vi "Process.vi"(8 "error in":errorcluster, 11 "Measurement.WavelengthSweeping.UI":refnum<class "Measurement.PhotocurrentMapping.UI.lvclass">) -> (0 "error out":errorcluster, 3 "Measurement.WavelengthSweeping.UI out":refnum<class "Measurement.PhotocurrentMapping.UI.lvclass">)   [LabVIEW 2017, in "Measurement.PhotocurrentMapping.UI.lvclass"]
doc: "---------------------------------------------------------------\nJKI State Machine Objects™\nhttp://jki.net/state-machine-objects/\nCopyright (C) 2005-2015, JKI <info@jki.net>\nALL RIGHTS RESERVEDJKI State Machine Objects (SMO) 1.0.0.5\nJKI - JKI\nCopyright (c) 2016, JKI"
uses:
  Measurement.PhotocurrentMapping.UI.lvclass
  D:/Program Files (x86)/National Instruments/LabVIEW 2017/vi.lib/JKI/JKI SMO/SMO/SMO.lvclass
  D:/Program Files (x86)/National Instruments/LabVIEW 2017/vi.lib/JKI/JKI SMO/SMO.UI/SMO.UI.lvclass
  <vilib>/JKI/JKI SMO/SMO/Typedefs/Parent Call--Enum.ctl
  Measurement.PhotocurrentMapping/Typedefs/Measurement.PhotocurrentMapping.Configured--Data.ctl
  Measurement.PhotocurrentMapping/Typedefs/Measurement.PhotocurrentMapping.Measured--Data.ctl
  Typedefs/Grid Data--Cluster.ctl
  Typedefs/Image Data--Cluster.ctl
  Typedefs/Graphs Data--Cluster.ctl
  <vilib>/vision/Image Controls.llb/IMAQ Image.ctl
  Measurement.PhotocurrentMapping/Measurement.PhotocurrentMapping.lvclass
  D:/upwork/Laser Measurement Tool/Laser/project/Subsystems/Measurement/Measurement.lvclass
  Measurement.UI/Measurement.UI.lvclass
  <vilib>/JKI/JKI SMO/SMO/SMO.lvclass
  <vilib>/JKI/JKI SMO/SMO.UI/SMO.UI.lvclass
  Measurement/Measurement.lvclass
panel:
  in  "Clear Button":bool
  in  "Stop Button":bool
  in  "Pause Button":bool
  in  "Start Button":bool
  in  "Close Button":bool
  in  "LIA Auto Scale":bool=TRUE
  in  "SMU Auto Scale":bool=TRUE
  in  "LIA maximum":dbl=1.0 min=0.0 step=0.01 format="%.4f"
  in  "LIA minimum":dbl min=0.0 step=0.01 format="%.4f"
  in  "SMU maximum, A":dbl=1.0 min=0.0 step=0.01 format="%.4f"
  in  "SMU minimum, A":dbl min=0.0 step=0.01 format="%.4f"
  out "Initialized":bool
  out "SMU":T1(plugin-control)
  out "LIA":T1(plugin-control)
  out "SMU":cluster{"X":dbl, "Y":dbl}[](graph) caption="XY Graph - Light"
  out "LIA":cluster{"X":dbl, "Y":dbl}[](graph) caption="XY Graph - Light"
  # "For instructions on how to use the JKI State Machine Objects, examples and video tutorials, visit:\nhttp://jki.net/state-machine-objects/\n\nJKI State Machine Objects™\nhttp://jki.net/state-machine-objects/\nCopyright (C) 2005-2015, JKI <info@jki.net>\nALL RIGHTS RESERVED"
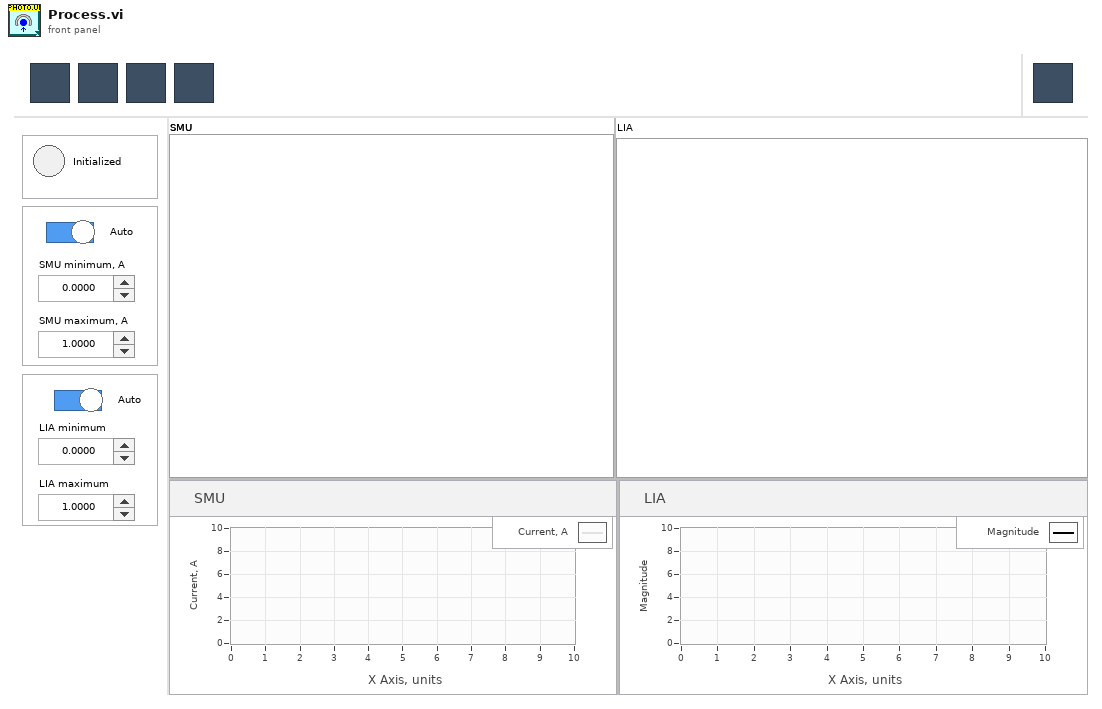
[diagram p1: front panel]
types:
  T1 = typedef "IMAQ Image.ctl" = refnum<image>
  T2 = typedef "SMO.lvclass/Parent Call--Enum.ctl" = enum16{"Allows parent to run", "Does not request parent to run"}
  T3 = enum8{"Enabled", "Disabled", "Disabled and Grayed Out"}
  T4 = enum32{"invalid app kind", "Development System", "Run Time System", "Student Edition", "Embedded LabVIEW", "Evaluation", "Custom"}
  T5 = enum32{"Invalid", "Standard", "Closed", "Hidden", "Minimized", "Maximized"}
  T6 = typedef "Measurement.lvclass/PublicEvents--Measurement.Initialized.ctl" = bool
  T7 = typedef "Measurement.PhotocurrentMapping.lvclass/Measurement.PhotocurrentMapping.Configured--Data.ctl" = cluster{"X Count":i32, "Y Count":i32}
  T8 = typedef "Measurement.lvclass/PublicEvents--Measurement.Configured.ctl" = variant
  T9 = typedef "Measurement.PhotocurrentMapping.UI.lvclass/Dependencies--Cluster.ctl" = cluster{"Measurement.PhotocurrentMapping":refnum<class "Measurement.PhotocurrentMapping.lvclass">}
  T10 = typedef "Measurement.PhotocurrentMapping.lvclass/Measurement.PhotocurrentMapping.Measured--Data.ctl" = cluster{"X Value, units":dbl, "Y Value, units":dbl, "X Index":i32, "Y Index":i32, "Current, A":dbl, "Magnitude":dbl, "Last Row Element?":bool}
  T11 = typedef "Measurement.PhotocurrentMapping.UI.lvclass/Grid Data--Cluster.ctl" = cluster{"SMU Image":T12, "LIA Image":T12, "Filled Row":i32}
  T12 = typedef "Measurement.PhotocurrentMapping.UI.lvclass/Image Data--Cluster.ctl" = cluster{"Raw":dbl[][], "Normalized":dbl[][], "Minimum":dbl, "Maximum":dbl}
  T13 = typedef "Measurement.PhotocurrentMapping.UI.lvclass/Graphs Data--Cluster.ctl" = cluster{"SMU Data":cluster{"X":dbl, "Y":dbl}[], "LIA Data":cluster{"X":dbl, "Y":dbl}[], "SMU Buffer":cluster{"X":dbl, "Y":dbl}[], "LIA Buffer":cluster{"X":dbl, "Y":dbl}[]}
  T14 = cluster{"Core":cluster{"Current VI Reference":refnum<vi>, "Close Panel on Exit?":bool, "error":errorcluster}, "Self Reference":refnum<class "Measurement.PhotocurrentMapping.UI.lvclass">, "Dependencies":T9, "Measured":T10, "X Count":i32, "Y Count":i32, "Grid Data":T11, "Graphs Data":T13, "SMU Image":T1, "LIA Image":T1}
  T15 = typedef "Measurement.lvclass/PublicEvents--Measurement.Measured.ctl" = variant
  T16 = typedef "Measurement.lvclass/PublicEvents--Measurement.Finished.ctl" = bool
  T17 = cluster{"Current VI Reference":refnum<vi>, "Close Panel on Exit?":bool, "error":errorcluster}
  T18 = typedef "Image Type" = u32
  T19 = typedef "SMO.lvclass/Protected Events.ctl" = cluster{"StopProcesses":refnum<user-event>, "AbortProcesses":refnum<user-event>, "Config Changed":refnum<user-event>, "Dependency":refnum<user-event>}
  T20 = cluster{"Event Registration Refnum":refnum<event-registration>, "Measurement Public Events":refnum<event-registration>}
  T21 = cluster{"X Value, units":dbl, "Current, A":dbl}[]
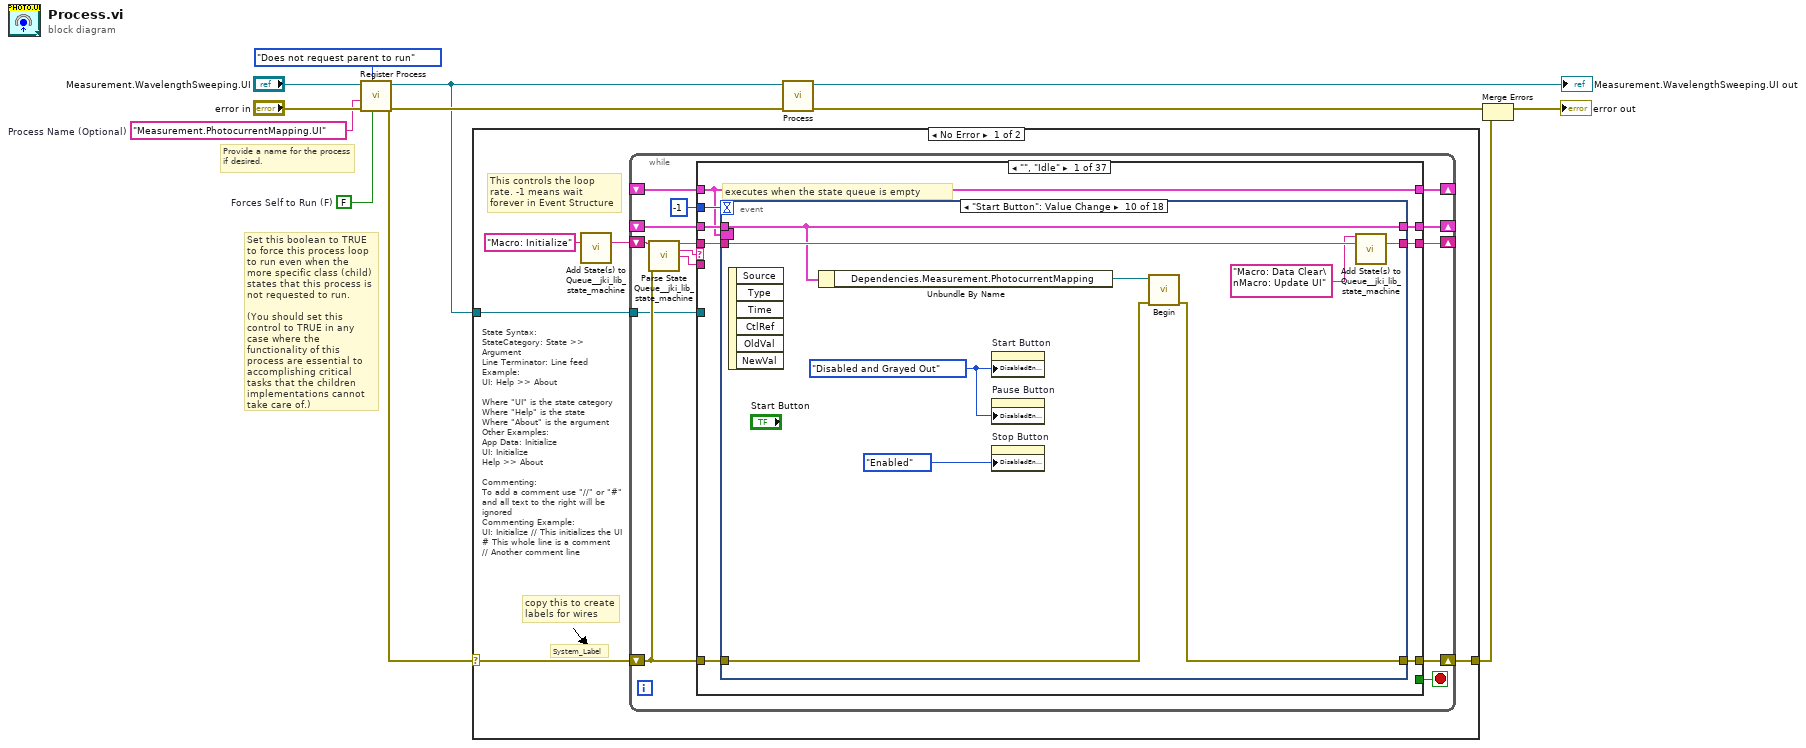
[diagram p0: block diagram]
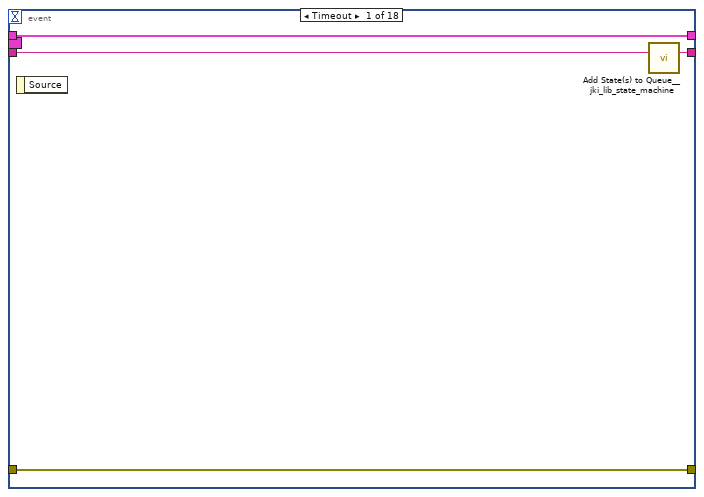
[diagram p2: hidden frame]
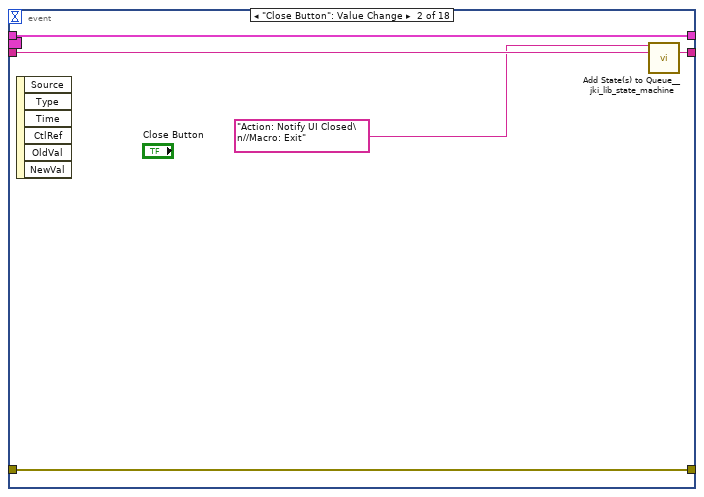
[diagram p3: hidden frame]
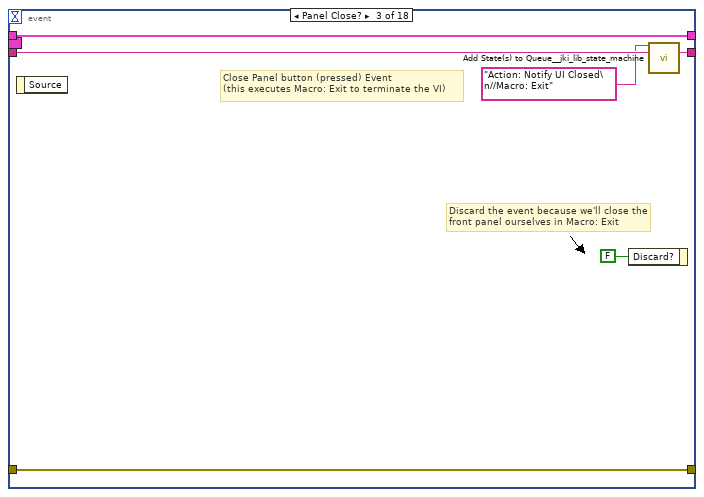
[diagram p4: hidden frame]
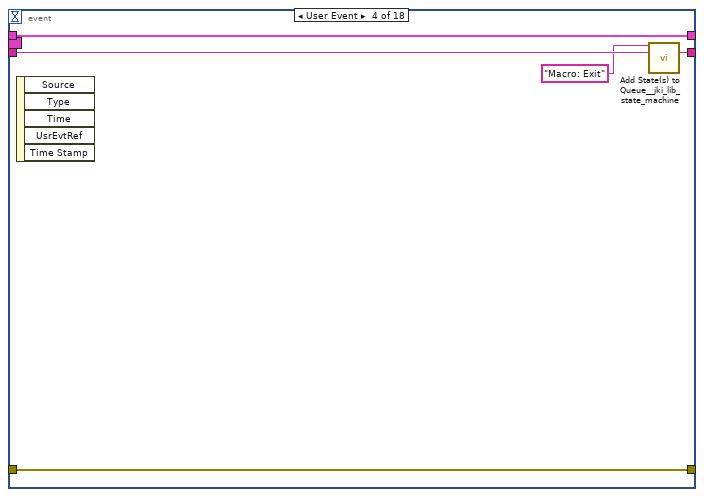
[diagram p5: hidden frame]
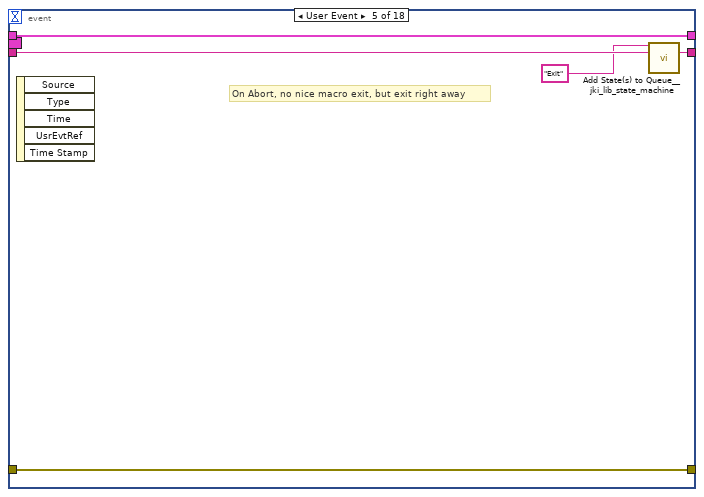
[diagram p6: hidden frame]
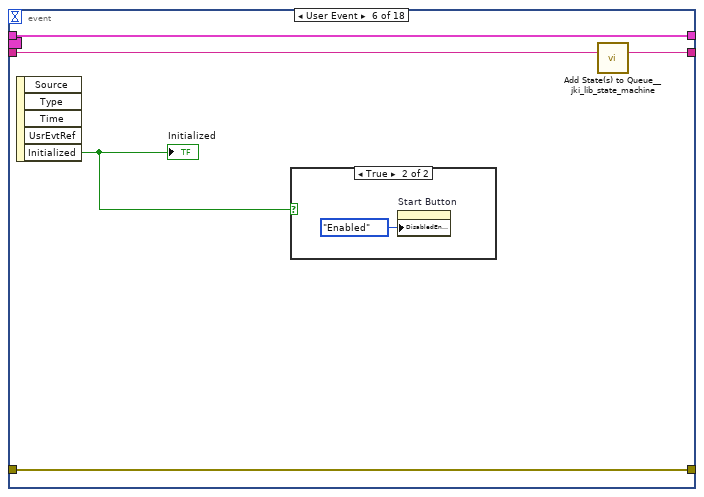
[diagram p7: hidden frame]
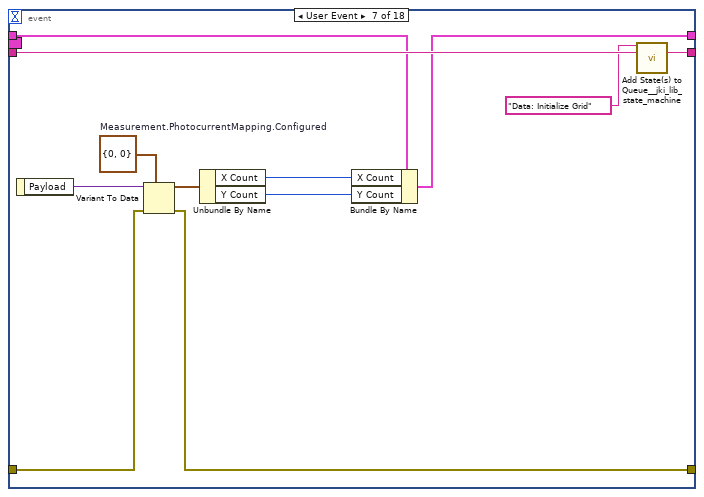
[diagram p9: hidden frame]
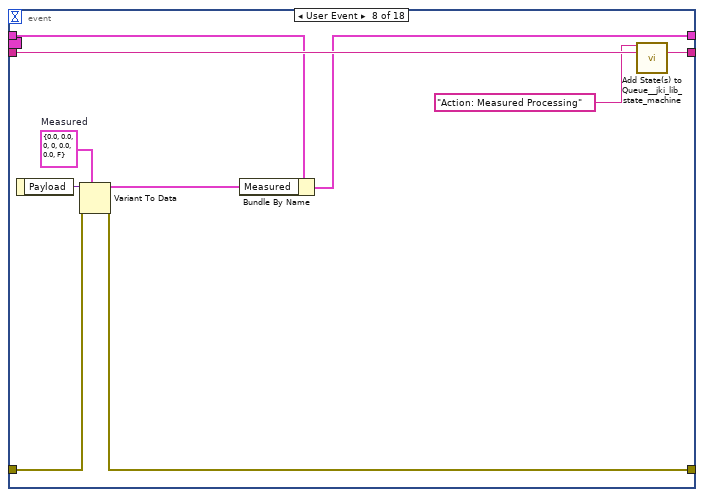
[diagram p10: hidden frame]
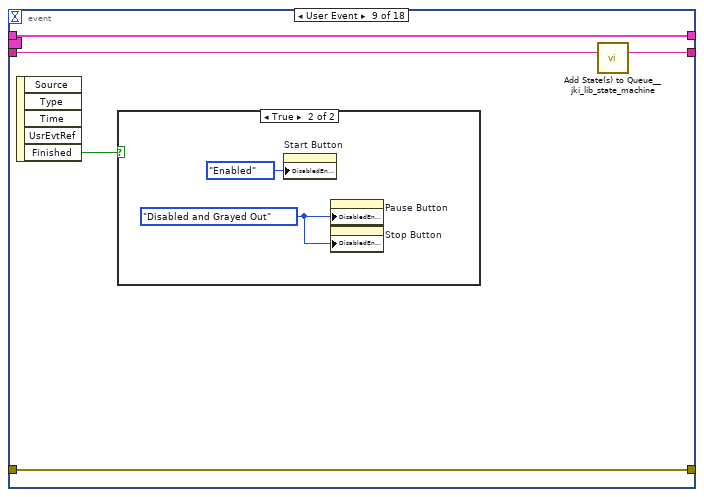
[diagram p11: hidden frame]
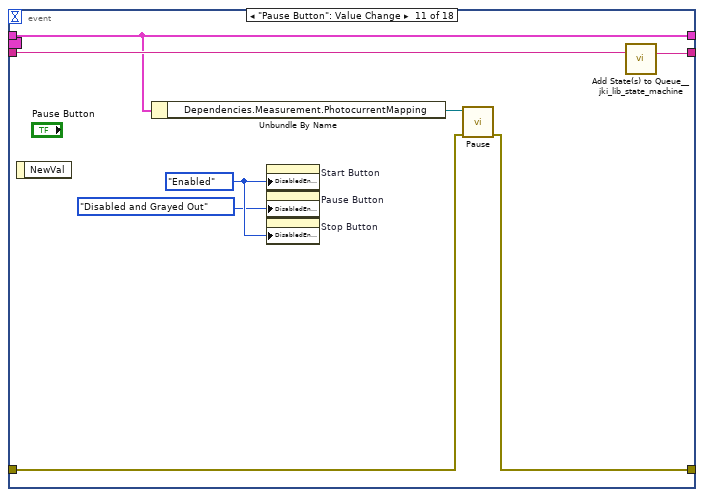
[diagram p13: hidden frame]
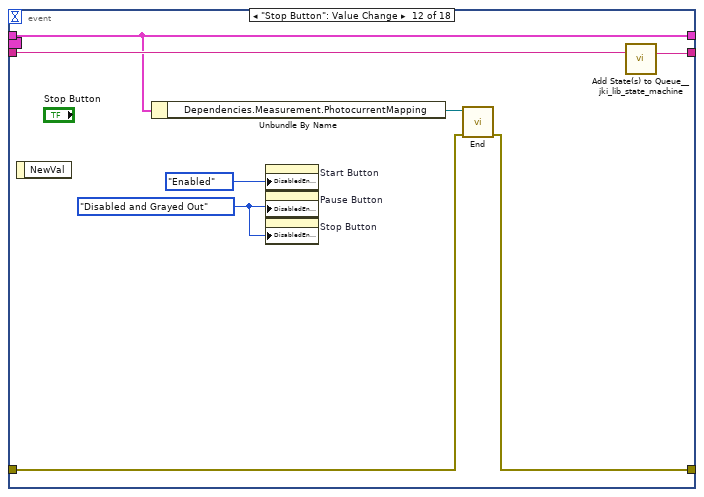
[diagram p14: hidden frame]
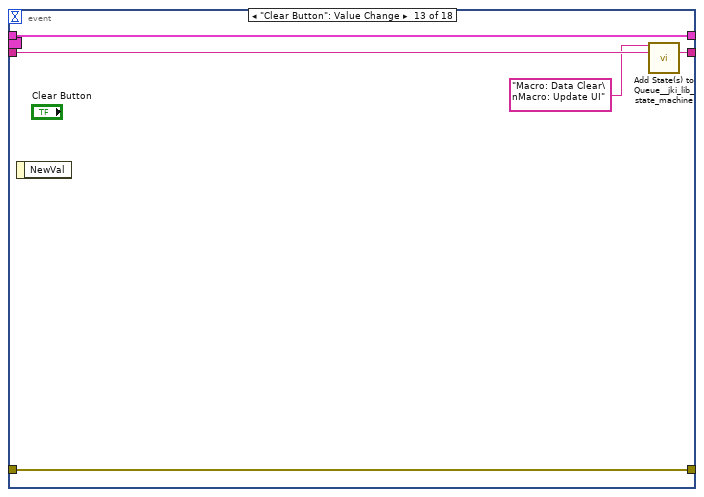
[diagram p15: hidden frame]
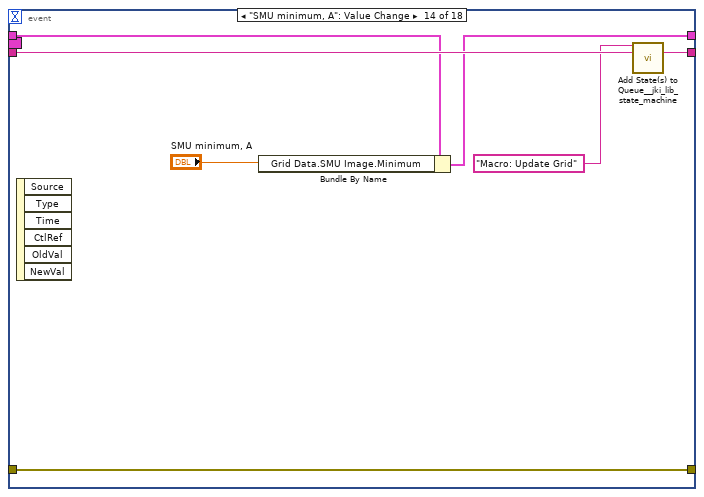
[diagram p16: hidden frame]
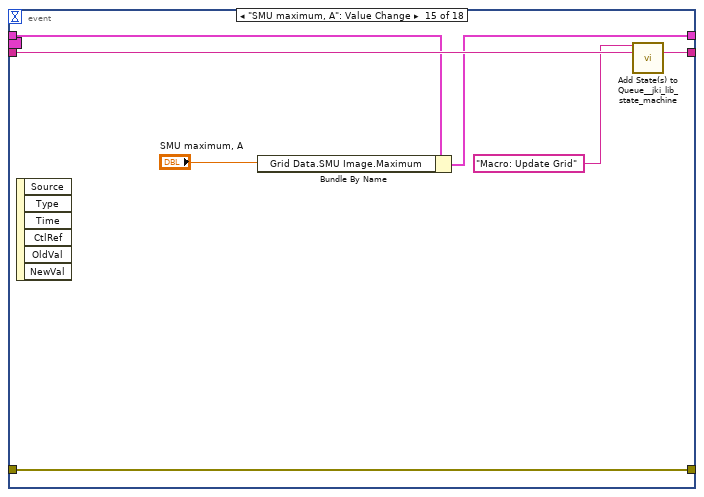
[diagram p17: hidden frame]
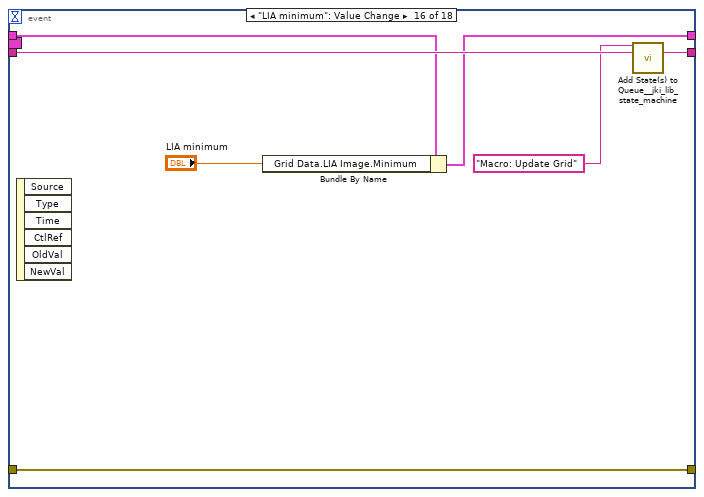
[diagram p18: hidden frame]
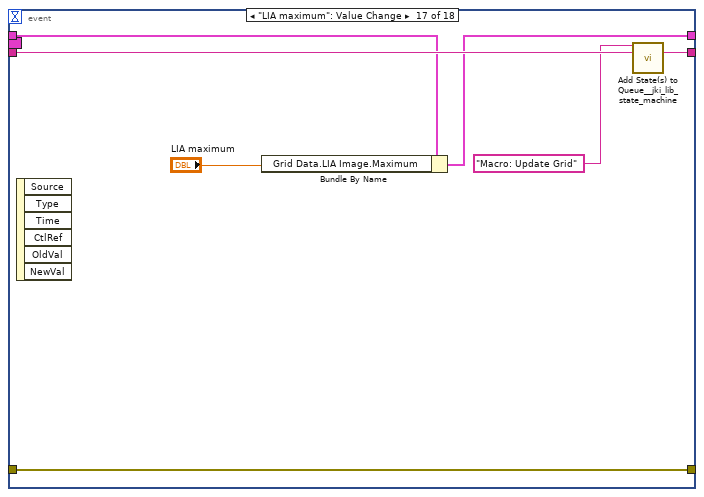
[diagram p19: hidden frame]
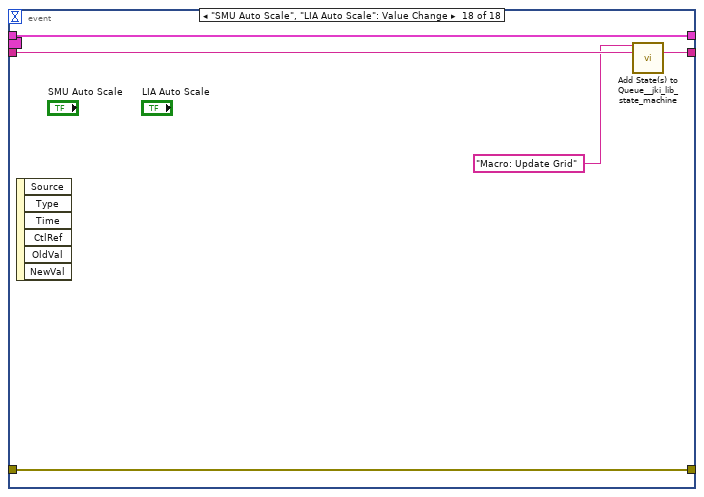
[diagram p20: hidden frame]
diagram:
  w2 = FALSE  # Forces Self to Run (F)
  w1 = "Measurement.PhotocurrentMapping.UI"  # Process Name (Optional)
  # "Provide a name for the process\nif desired."
  # "Set this boolean to TRUE to force this process loop to run even when the more specific class (child) states that this process is not requested to run.\n\n(You should set this control to TRUE in any case where the functionality of this process are essential to accomplishing critical tasks that the children implementations cannot take care of.)"
  n1 = call <vilib>:"Register Process.vi"("Forces Self to Run (F)"=w2, "Parent Call"=Parent_Call--Enum."Does not request parent to run", "error in (no error)"="error in", "Process Name (optional)"=w1, "SMO"="Measurement.WavelengthSweeping.UI") -> ("error out"=w8:errorcluster, "SMO out"=w7:refnum<class "Measurement.PhotocurrentMapping.UI.lvclass">)  [unwired: 5 in]
  n2 = case shown="No Error" w8 {
    selector: w8 -> [w13 w573]
    tunnel: w7 -> [w14 _]
    tunnel: [w12 w573] -> w4
    frame No Error {
      # "State Syntax:\nStateCategory: State >> Argument\nLine Terminator: Line feed\nExample:\nUI: Help >> About\n\nWhere \"UI\" is the state category\nWhere \"Help\" is the state\nWhere \"About\" is the argument\nOther Examples:\nApp Data: Initialize\nUI: Initialize\nHelp >> About\n\nCommenting:\nTo add a comment use \"//\" or \"#\" and all text to the right will be ignored\nCommenting Example:\nUI: Initialize // This initializes the UI\n# This whole line is a comment\n// Another comment line"
      # "copy this to create labels for wires"
      # "This controls the loop rate. -1 means wait forever in Event Structure"
      # "System_Label"
      n3 = call <vilib>:"Add State(s) to Queue__jki_lib_state_machine.vi"("State(s) in (\"\")"="Macro: Initialize") -> ("States Out"=w16:string)  [unwired: 14 in]
      n4 = while {
        shift-right: [w23] -> _
        shift-left: _ -> [w22]
        shift-right: [w26] -> w12
        shift-left: w13 -> [w20]
        shift-right: [w25] -> _
        shift-left: w16 -> [w27]
        tunnel: w14 -> [w19]
        shift-right: [w18] -> _
        shift-left: _ -> [w17]
        stop <- w24 stop-if-true
        n5 = call <vilib>:"Parse State Queue__jki_lib_state_machine.vi"("State Queue"=w27, "Error In (no error)"=w20) -> ("Remaining States"=w29:string, "Current State"=w30:string, "Arguments"=w28:string)  [unwired: 11 in]
        n6 = case shown="\"\", \"Idle\"" w30 {
          selector: w30 -> [_ _ w168 _ _ _ _ _ _ _ _ _ _ _ _ _ _ _ _ _ _ _ _ _ _ _ _ _ _ _ _ _ _ _ _ _ _]
          tunnel: w29 -> [w38 w166 w172 w191 w205 w211 w216 w235 w242 w253 w259 w272 w277 w292 w299 w315 w349 w356 w361 w370 w384 w390 w396 w402 w407 w418 w423 w437 w443 w450 w457 w463 w481 w512 w527 w557 w572]
          tunnel: w28 -> [_ _ _ _ _ _ _ _ _ _ _ _ _ _ w293 w309 _ _ _ _ _ _ _ _ _ _ _ _ _ _ _ _ _ _ _ _ _]
          tunnel: w22 -> [w36 w163 w170 w182 w194 w207 w213 _ w237 w247 w257 w266 w274 w288 w297 w311 w345 w352 w358 w366 w375 w387 w393 w399 w404 w415 w420 w429 w441 w446 w453 w458 w476 w507 w518 w542 w563]
          tunnel: [w35 w164 w174 w188 w196 w206 w214 w224 w238 w250 w258 w269 w275 w278 w294 w312 w346 w353 w359 w368 w382 w388 w394 w400 w405 w409 w421 w431 w438 w447 w451 w460 w478 w509 w524 w554 w560] -> w26
          tunnel: w20 -> [w34 w164 w173 w188 w201 _ w214 w232 w239 w250 w258 w269 w275 w280 w295 w313 w346 w353 w359 w368 w382 w388 w394 w400 w405 w410 w421 w433 w439 w447 w452 w460 w478 w509 w524 w554 w561]
          tunnel: [w37 w165 w171 w190 w204 w210 w215 w234 w241 w252 w260 w271 w276 w291 w298 w314 w348 w355 w360 w369 w383 w389 w395 w401 w406 w417 w422 w436 w442 w449 w456 w462 w480 w511 w526 w556 w571] -> w25
          tunnel: [_ _ _ _ _ TRUE _ _ _ _ _ _ _ _ _ _ _ _ _ _ _ _ _ _ _ _ _ _ _ _ _ _ _ _ _ _ _] -> w24
          tunnel: [w33 w163 w170 w189 w193 w207 w213 w233 w237 w246 w256 w265 w274 w287 w297 w311 w345 w352 w358 w366 w375 w387 w393 w399 w404 w415 w420 w429 w441 w445 w453 w458 w475 w506 w523 w553 w566] -> w23
          tunnel: -1 ("Timeout") -> [w32 _ _ _ _ _ _ _ _ _ _ _ _ _ _ _ _ _ _ _ _ _ _ _ _ _ _ _ _ _ _ _ _ _ _ _ _]
          tunnel: w19 -> [_ _ _ _ _ _ _ w230 _ _ _ _ _ _ _ _ _ _ _ _ _ _ _ _ _ _ _ _ _ _ _ _ _ _ _ _ _]
          tunnel: [w31 w162 w167 w179 w203 w208 w212 w229 w236 w251 w261 w270 w273 w290 w296 w308 w347 w354 w357 w367 w376 w386 w392 w398 w403 w416 w419 w426 w440 w448 w455 w461 w479 w510 w525 w555 w570] -> w18
          tunnel: w17 -> [w31 w162 w167 w179 w203 w208 w212 w229 w236 w251 w261 w270 w273 w290 w296 w308 w347 w354 w357 w367 w376 w386 w392 w398 w403 w416 w419 _ w440 w448 w455 w461 w479 w510 w525 w555 w570]
          frame "", "Idle" {
            # "executes when the state queue is empty"
            n7 = event shown="[9] \"Start Button\": Value Change" {
              selector: w31 -> [_ _ _ _ _ _ _ _ _ _ _ _ _ _ _ _ _ _]
              dyn-events: _ -> [_ _ _ _ _ _ _ _ _ _ _ _ _ _ _ _ _ _]
              timeout: w32 -> [_ _ _ _ _ _ _ _ _ _ _ _ _ _ _ _ _ _]
              tunnel: w38 -> [w42 w47 w53 w58 w63 w65 w80 w90 w93 w106 w114 w122 w128 w133 w140 w147 w154 w159]
              tunnel: [w41 w46 w52 w57 w62 w66 w81 w91 w94 w107 w115 w123 w127 w134 w141 w148 w155 w160] -> w37
              tunnel: w36 -> [w39 w44 w49 w55 w60 w67 w74 w84 w95 w105 w113 w121 w125 w132 w139 w146 w153 w158]
              tunnel: [w40 w45 w48 w56 w61 w68 w78 w85 w96 w102 w110 w118 w126 w135 w142 w149 w156 w161] -> w35
              tunnel: w34 -> [w40 w45 w48 w56 w61 w68 w79 w89 w96 w103 w111 w119 w126 w135 w142 w149 w156 w161]
              tunnel: [w39 w44 w49 w55 w60 w67 w73 w83 w95 w105 w113 w121 w125 w131 w138 w145 w152 w158] -> w33
              event Timeout {
                n8 = event-data() -> ()  [unwired: 1 in, 1 out]
                n9 = call <vilib>:"Add State(s) to Queue__jki_lib_state_machine.vi"("State(s) in (\"\")"=w42) -> ("States Out"=w41:string)  [unwired: 14 in]
              }
              event "Close Button": Value Change {
                n10 = event-data() -> ()  [unwired: 1 in, 6 out]
                n11 = call <vilib>:"Add State(s) to Queue__jki_lib_state_machine.vi"("State(s) in Front (\"\")"="Action: Notify UI Closed\n//Macro: Exit" ("State(s) in Front (\"\")"), "State(s) in (\"\")"=w47) -> ("States Out"=w46:string)  [unwired: 13 in]
              }
              event Panel Close? {
                # "Discard the event because we'll close the front panel ourselves in Macro: Exit"
                # "Close Panel button (pressed) Event\n(this executes Macro: Exit to terminate the VI)"
                n12 = event-data() -> ()  [unwired: 1 in, 1 out]
                n13 = event-data("Discard?"=FALSE) -> ()  [unwired: 1 in, 1 out]
                n14 = call <vilib>:"Add State(s) to Queue__jki_lib_state_machine.vi"("State(s) in Front (\"\")"="Action: Notify UI Closed\n//Macro: Exit", "State(s) in (\"\")"=w53) -> ("States Out"=w52:string)  [unwired: 13 in]
              }
              event User Event {
                n15 = event-data() -> ()  [unwired: 1 in, 5 out]
                n16 = call <vilib>:"Add State(s) to Queue__jki_lib_state_machine.vi"("State(s) in Front (\"\")"="Macro: Exit", "State(s) in (\"\")"=w58) -> ("States Out"=w57:string)  [unwired: 13 in]
              }
              event User Event {
                # "On Abort, no nice macro exit, but exit right away"
                n17 = event-data() -> ()  [unwired: 1 in, 5 out]
                n18 = call <vilib>:"Add State(s) to Queue__jki_lib_state_machine.vi"("State(s) in Front (\"\")"="Exit", "State(s) in (\"\")"=w63) -> ("States Out"=w62:string)  [unwired: 13 in]
              }
              event User Event {
                n19 = event-data() -> ("Initialized"=w64:T6)  [unwired: 1 in, 4 out]
                "Initialized" <- w64
                n20 = case shown="True" w64 {
                  frame False {
                  }
                  frame True {
                    n21 = property on="Start Button" class="Bool"("DisabledEnum"=T3."Enabled" ("Disabled")) -> ()  [unwired: 2 in, 2 out]
                  }
                }
                n22 = call <vilib>:"Add State(s) to Queue__jki_lib_state_machine.vi"("State(s) in (\"\")"=w65) -> ("States Out"=w66:string)  [unwired: 14 in]
              }
              event User Event {
                w76 = T7 {"X Count"=0, "Y Count"=0}  # Measurement.PhotocurrentMapping.Configured
                n23 = event-data() -> ("Payload"=w77:T8)  [unwired: 1 in]
                n24 = Variant To Data(error in=w79, type=w76, Variant=w77) -> (data=w75:T7, error out=w78:errorcluster)
                n25 = Unbundle By Name(w75) -> ("X Count"=w72:i32, "Y Count"=w71:i32)
                n26 = Bundle By Name(cluster=w74, "X Count"=w72, "Y Count"=w71) -> (w73:T14)
                n27 = call <vilib>:"Add State(s) to Queue__jki_lib_state_machine.vi"("State(s) in Front (\"\")"="Data: Initialize Grid", "State(s) in (\"\")"=w80) -> ("States Out"=w81:string)  [unwired: 13 in]
              }
              event User Event {
                w87 = T10 {"X Value, units"=0.0, "Y Value, units"=0.0, "X Index"=0, "Y Index"=0, "Current, A"=0.0, "Magnitude"=0.0, "Last Row Element?"=FALSE}  # Measured
                n28 = event-data() -> ("Payload"=w88:T15)  [unwired: 1 in]
                n29 = Variant To Data(error in=w89, type=w87, Variant=w88) -> (data=w82:T10, error out=w85:errorcluster)
                n30 = Bundle By Name(cluster=w84, "Measured"=w82) -> (w83:T14)
                n31 = call <vilib>:"Add State(s) to Queue__jki_lib_state_machine.vi"("State(s) in Front (\"\")"="Action: Measured Processing", "State(s) in (\"\")"=w90) -> ("States Out"=w91:string)  [unwired: 13 in]
              }
              event User Event {
                n32 = event-data() -> ("Finished"=w92:T16)  [unwired: 1 in, 4 out]
                n33 = case shown="True" w92 {
                  frame False {
                  }
                  frame True {
                    w97 = T3."Disabled and Grayed Out" ("Disabled")
                    n34 = property on="Start Button" class="Bool"("DisabledEnum"=T3."Enabled" ("Disabled")) -> ()  [unwired: 2 in, 2 out]
                    n35 = property on="Pause Button" class="Bool"("DisabledEnum"=w97) -> ()  [unwired: 2 in, 2 out]
                    n36 = property on="Stop Button" class="Bool"("DisabledEnum"=w97) -> ()  [unwired: 2 in, 2 out]
                  }
                }
                n37 = call <vilib>:"Add State(s) to Queue__jki_lib_state_machine.vi"("State(s) in (\"\")"=w93) -> ("States Out"=w94:string)  [unwired: 14 in]
              }
              event "Start Button": Value Change {
                w100 = T3."Disabled and Grayed Out" ("Disabled")
                n38 = event-data() -> ()  [unwired: 1 in, 6 out]
                n39 = Unbundle By Name(w105) -> ("Dependencies.Measurement.PhotocurrentMapping"=w104:refnum<class "Measurement.PhotocurrentMapping.lvclass">)
                n40 = property on="Start Button" class="Bool"("DisabledEnum"=w100) -> ()  [unwired: 2 in, 2 out]
                n41 = property on="Pause Button" class="Bool"("DisabledEnum"=w100) -> ()  [unwired: 2 in, 2 out]
                n42 = property on="Stop Button" class="Bool"("DisabledEnum"=T3."Enabled" ("Disabled")) -> ()  [unwired: 2 in, 2 out]
                n43 = call "Begin.vi"("error in (no error)"=w103, "Measurement in"=w104) -> ("error out"=w102:errorcluster)  [unwired: 8 in, 1 out]
                n44 = call <vilib>:"Add State(s) to Queue__jki_lib_state_machine.vi"("State(s) in Front (\"\")"="Macro: Data Clear\nMacro: Update UI", "State(s) in (\"\")"=w106) -> ("States Out"=w107:string)  [unwired: 13 in]
              }
              event "Pause Button": Value Change {
                w109 = T3."Enabled" ("Disabled")
                n45 = event-data() -> ()  [unwired: 1 in, 1 out]
                n46 = Unbundle By Name(w113) -> ("Dependencies.Measurement.PhotocurrentMapping"=w112:refnum<class "Measurement.PhotocurrentMapping.lvclass">)
                n47 = property on="Start Button" class="Bool"("DisabledEnum"=w109) -> ()  [unwired: 2 in, 2 out]
                n48 = property on="Pause Button" class="Bool"("DisabledEnum"=T3."Disabled and Grayed Out" ("Disabled")) -> ()  [unwired: 2 in, 2 out]
                n49 = property on="Stop Button" class="Bool"("DisabledEnum"=w109) -> ()  [unwired: 2 in, 2 out]
                n50 = call "Pause.vi"("error in (no error)"=w111, "Measurement in"=w112) -> ("error out"=w110:errorcluster)  [unwired: 8 in, 1 out]
                n51 = call <vilib>:"Add State(s) to Queue__jki_lib_state_machine.vi"("State(s) in (\"\")"=w114) -> ("States Out"=w115:string)  [unwired: 14 in]
              }
              event "Stop Button": Value Change {
                w116 = T3."Disabled and Grayed Out" ("Disabled")
                n52 = event-data() -> ()  [unwired: 1 in, 1 out]
                n53 = Unbundle By Name(w121) -> ("Dependencies.Measurement.PhotocurrentMapping"=w120:refnum<class "Measurement.PhotocurrentMapping.lvclass">)
                n54 = property on="Start Button" class="Bool"("DisabledEnum"=T3."Enabled" ("Disabled")) -> ()  [unwired: 2 in, 2 out]
                n55 = property on="Pause Button" class="Bool"("DisabledEnum"=w116) -> ()  [unwired: 2 in, 2 out]
                n56 = property on="Stop Button" class="Bool"("DisabledEnum"=w116) -> ()  [unwired: 2 in, 2 out]
                n57 = call "End.vi"("error in (no error)"=w119, "Measurement in"=w120) -> ("error out"=w118:errorcluster)  [unwired: 8 in, 1 out]
                n58 = call <vilib>:"Add State(s) to Queue__jki_lib_state_machine.vi"("State(s) in (\"\")"=w122) -> ("States Out"=w123:string)  [unwired: 14 in]
              }
              event "Clear Button": Value Change {
                n59 = event-data() -> ()  [unwired: 1 in, 1 out]
                n60 = call <vilib>:"Add State(s) to Queue__jki_lib_state_machine.vi"("State(s) in Front (\"\")"="Macro: Data Clear\nMacro: Update UI", "State(s) in (\"\")"=w128) -> ("States Out"=w127:string)  [unwired: 13 in]
              }
              event "SMU minimum, A": Value Change {
                n61 = event-data() -> ()  [unwired: 1 in, 6 out]
                n62 = Bundle By Name(cluster=w132, "Grid Data.SMU Image.Minimum"="SMU minimum, A") -> (w131:T14)
                n63 = call <vilib>:"Add State(s) to Queue__jki_lib_state_machine.vi"("State(s) in Front (\"\")"="Macro: Update Grid" ("State(s) in Front (\"\")"), "State(s) in (\"\")"=w133) -> ("States Out"=w134:string)  [unwired: 13 in]
              }
              event "SMU maximum, A": Value Change {
                n64 = event-data() -> ()  [unwired: 1 in, 6 out]
                n65 = Bundle By Name(cluster=w139, "Grid Data.SMU Image.Maximum"="SMU maximum, A") -> (w138:T14)
                n66 = call <vilib>:"Add State(s) to Queue__jki_lib_state_machine.vi"("State(s) in Front (\"\")"="Macro: Update Grid" ("State(s) in Front (\"\")"), "State(s) in (\"\")"=w140) -> ("States Out"=w141:string)  [unwired: 13 in]
              }
              event "LIA minimum": Value Change {
                n67 = event-data() -> ()  [unwired: 1 in, 6 out]
                n68 = Bundle By Name(cluster=w146, "Grid Data.LIA Image.Minimum"="LIA minimum") -> (w145:T14)
                n69 = call <vilib>:"Add State(s) to Queue__jki_lib_state_machine.vi"("State(s) in Front (\"\")"="Macro: Update Grid" ("State(s) in Front (\"\")"), "State(s) in (\"\")"=w147) -> ("States Out"=w148:string)  [unwired: 13 in]
              }
              event "LIA maximum": Value Change {
                n70 = event-data() -> ()  [unwired: 1 in, 6 out]
                n71 = Bundle By Name(cluster=w153, "Grid Data.LIA Image.Maximum"="LIA maximum") -> (w152:T14)
                n72 = call <vilib>:"Add State(s) to Queue__jki_lib_state_machine.vi"("State(s) in Front (\"\")"="Macro: Update Grid" ("State(s) in Front (\"\")"), "State(s) in (\"\")"=w154) -> ("States Out"=w155:string)  [unwired: 13 in]
              }
              event "SMU Auto Scale", "LIA Auto Scale": Value Change {
                n73 = event-data() -> ()  [unwired: 1 in, 6 out]
                n74 = call <vilib>:"Add State(s) to Queue__jki_lib_state_machine.vi"("State(s) in Front (\"\")"="Macro: Update Grid" ("State(s) in Front (\"\")"), "State(s) in (\"\")"=w159) -> ("States Out"=w160:string)  [unwired: 13 in]
              }
            }
          }
          frame "---------- Core ----------" {
            # "Do not put any code in this frame.\n(it is a separator no-op)"
            n75 = call <vilib>:"Add State(s) to Queue__jki_lib_state_machine.vi"("State(s) in (\"\")"=w166) -> ("States Out"=w165:string)  [unwired: 14 in]
          }
          frame Default {
            w177 = 42 items=["No error", "Argument error", "Memory is full", "Out of zone", "End of file", "File already open", "Generic file I/O error", "File not found", "File permission error", "Disk is full", "Duplicate path", "Too many files open", "System feature not enabled", "Resource file not found", "Cannot add resource", "Resource not found", "Image not found", "Image memory error", "Pen does not exist", "Config type invalid", "Config token not found", "Config parse error", "Config memory error", "Bad external code format", "Bad external code offset", "External code not present", "Null window", "Destroy window error", "Null menu", "Print aborted", "Bad print record", "Print driver error", "Windows error during printing", "Memory error during printing", "Print dialog error", "Generic print error", "Invalid device refnum", "Device not found", "Device parameter error", "Device unit error", "Cannot open device", "Device call aborted", "Generic error", "Cancelled by user", "Object ID too low", "Object ID too high", "Object not in heap", "Unknown heap", "Unknown object (invalid DefProc)", "Unknown object (DefProc not in table)", "Message out of range", "Invalid (null) method", "Unknown message", "Manager call not supported", "Bad address", "Network operation in progress", "Network operation timed out", "Connection is busy", "Network attribute not supported", "Network error", "Address in use", "System out of memory", "Connection aborted", "Connection refused", "Not connected", "Already connected", "Connection closed", "Initialization error (interapplication manager)", "Bad occurrence", "Wait on unbound occurrence handler", "Occurrence queue overflow", "Datalog type conflict", "Unused", "Unrecognized type (interapplication manager)", "Memory corrupt", "Failed to make temporary DLL", "Old CIN version", "Drag socket not found", "Failed to load drop-object", "Failed to register OLE object", "Failed to release OLE object", "Format specifier type mismatch", "Unknown format specifier", "Too few format specifiers", "Too many format specifiers", "Scan failed", "Newer CIN version", "Error converting to variant", "Runtime menu error", "Password tampered", "Variant attribute not found", "Incompatible variant data type", "Event data is not available", "Event Store is not present", "Occurrence is not found", "Event Queue is not created", "Event info is not available", "Refnum passed is NULL", "Error retrieving Class GUID", "Error retrieving CoClass GUID", "Error retrieving TypeLib GUID.", "Bad built application magic bytes.", "Specific driver is different from the specific driver associated with the Logical Name.", "There is no session opened to the class driver.", "Max Error", "MAX - Error with config objects", "MAX - Error loading configuration", "MAX - Group not supported"]
            # "Current State"
            # "Do not delete, rename, or modify this frame.\n(this is used to capture unhandled states and typos)"
            # "Handle mistyped state name (developer tool)"
            n76 = Format Into String(format string="Software Exception: Unhandled State \"%s\"." ("message"), error in=w173, w168) -> (resulting string=w176:string, error out=w175:errorcluster)  [unwired: 1 in]
            n77 = call <vilib>:"Error Cluster From Error Code.vi"("show call chain? (False)"=TRUE, "error in (no error)"=w175, "error message (\"\")"=w176, "error code (0)"=w177) -> ("error out"=w174:errorcluster)  [unwired: 5 in]
            n78 = call <vilib>:"Add State(s) to Queue__jki_lib_state_machine.vi"("State(s) in (\"\")"=w172) -> ("States Out"=w171:string)  [unwired: 14 in]
          }
          frame "Initialize Core Data" {
            # "Do not delete, rename, or modify this frame.\n(this is used to determine panel behavior on exit)"
            # "originally closed?"
            # "exe?"
            # "If panel starts closed or is an EXE, then close it when we exit"
            n79 = property class="VI"() -> ("Front Panel.Open"=w187:bool)  [unwired: 2 in, 2 out]
            n80 = property class="App"() -> ("App.Kind"=w186:T4)  [unwired: 2 in, 2 out]
            n81 = control-ref of="Current VI Reference"() -> (w180:refnum<vi>)
            n82 = Not(x=w187) -> (.not. x?=w184:bool)
            n83 = Equal?(x=w186, y=T4."Run Time System" ("Application:Kind")) -> (x = y?=w183:bool)
            n84 = Or(x=w184, y=w183) -> (x .or. y?=w181:bool)
            n85 = Bundle By Name(cluster=w182, "Core.Current VI Reference"=w180, "Core.Close Panel on Exit?"=w181) -> (w189:T14)
            n86 = call <vilib>:"Add State(s) to Queue__jki_lib_state_machine.vi"("State(s) in (\"\")"=w191) -> ("States Out"=w190:string)  [unwired: 14 in]
          }
          frame "Error Handler" {
            w196 = errorcluster {"status"=FALSE, "code"=0, "source"=""}  # No error
            # "Overwrite this method to handle errors and pass to parent if not handled. Parent will fire a public event if the error is not handled up the chain of classes."
            # "Handle any errors here.\nYou can also output any states to clean-up after errors occur"
            n87 = Unbundle By Name(w194) -> ("Self Reference"=w202:refnum<class "Measurement.PhotocurrentMapping.UI.lvclass">)
            n88 = call-dynamic "Handle Error.vi"("Stop on Unhandled Error (T)"=TRUE, "error in"=w201, "SMO"=w202) -> ("handling error"=w197:errorcluster, "Unhandled error"=w195:errorcluster)  [unwired: 6 in, 1 out]
            n89 = Bundle By Name(cluster=w194, "Core.error"=w195) -> (w193:T14)
            n90 = Select(t="Exit", s=w197, f="") -> (s? t:f=w198:string)
            n91 = call <vilib>:"Add State(s) to Queue__jki_lib_state_machine.vi"("State(s) in Front (\"\")"=w198, "State(s) in (\"\")"=w205) -> ("States Out"=w204:string)  [unwired: 13 in]
          }
          frame "Exit" {
            # "Do not put any code in this frame.\n(No errors that occur here will be handled.)"
            n92 = Unbundle By Name(w207) -> ("Core.error"=w206:errorcluster)
            n93 = call <vilib>:"Add State(s) to Queue__jki_lib_state_machine.vi"("State(s) in (\"\")"=w211) -> ("States Out"=w210:string)  [unwired: 14 in]
          }
          frame "---------- Data ----------" {
            # "Do not put any code in this frame.\n(It is a separator no-op. You can make a copy of this frame to create a new Data frame)"
            n94 = call <vilib>:"Add State(s) to Queue__jki_lib_state_machine.vi"("State(s) in (\"\")"=w216) -> ("States Out"=w215:string)  [unwired: 14 in]
          }
          frame "Data: Initialize" {
            w217 = T1 refnum  # LIA Image
            w218 = T1 refnum  # SMU Image
            w222 = T13 {"SMU Data"=[], "LIA Data"=[], "SMU Buffer"=[], "LIA Buffer"=[]}  # Graphs Data
            w223 = T10 {"X Value, units"=0.0, "Y Value, units"=0.0, "X Index"=0, "Y Index"=0, "Current, A"=0.0, "Magnitude"=0.0, "Last Row Element?"=FALSE}  # Measured
            w220 = 0  # Y Count
            w221 = 0  # X Count
            w219 = T11 {"SMU Image"={"Raw"=[], "Normalized"=[], "Minimum"=0.0, "Maximum"=0.0}, "LIA Image"={"Raw"=[], "Normalized"=[], "Minimum"=0.0, "Maximum"=0.0}, "Filled Row"=0}  # Grid Data
            w228 = T17 {"Current VI Reference"=refnum, "Close Panel on Exit?"=FALSE, "error"={"status"=FALSE, "code"=0, "source"=""}}  # Core
            w231 = refnum<class "Measurement.PhotocurrentMapping.UI.lvclass"> refnum  # Self Reference
            # "do not delete - used by framework"
            # "Data names and types of shift register data are defined by this bundle."
            # "Initialize the shift-register data, here.\n(data names are defined by what you wire into the bundle function)"
            n95 = Variant To Data(error in=w232, type=w231, Variant=w230) -> (data=w227:refnum<class "Measurement.PhotocurrentMapping.UI.lvclass">, error out=w225:errorcluster)
            n96 = call "Measurement.WavelengthSweeping.UI.GetDependencies.vi"("error in (no error)"=w225, "Measurement.PhotocurrentMapping.UI in"=w227) -> ("error out"=w224:errorcluster, "Dependencies"=w226:T9)  [unwired: 7 in, 1 out]
            n97 = Bundle("Core"=w228, "Self Reference"=w227, "Dependencies"=w226, "Measured"=w223, "X Count"=w221, "Y Count"=w220, "Grid Data"=w219, "Graphs Data"=w222, "SMU Image"=w218, "LIA Image"=w217) -> (w233:T14)  [unwired: 1 in]
            n98 = call <vilib>:"Add State(s) to Queue__jki_lib_state_machine.vi"("State(s) in (\"\")"=w235) -> ("States Out"=w234:string)  [unwired: 14 in]
          }
          frame "Data: Cleanup" {
            # "Cleanup any data and references, here.\n(this is called automatically, by the Macro: Exit)"
            n99 = Unbundle By Name(w237) -> ("Core.Current VI Reference"=w240:refnum<vi>)
            n100 = Close Reference(reference=w240, error in (no error)=w239) -> (error out=w238:errorcluster)
            n101 = call <vilib>:"Add State(s) to Queue__jki_lib_state_machine.vi"("State(s) in (\"\")"=w242) -> ("States Out"=w241:string)  [unwired: 14 in]
          }
          frame "Data: Initialize Grid" {
            w249 = 0.0  # Initial Value
            n102 = Unbundle By Name(w247) -> ("X Count"=w243:i32, "Y Count"=w248:i32)
            n103 = Initialize Array(w249, w248, w243) -> (w245:dbl[][])
            n104 = Bundle By Name(cluster=w247, "Grid Data.SMU Image.Raw"=w245, "Grid Data.SMU Image.Normalized"=w245, "Grid Data.LIA Image.Raw"=w245, "Grid Data.LIA Image.Normalized"=w245, "Grid Data.Filled Row"=0) -> (w246:T14)
            n105 = call <vilib>:"Add State(s) to Queue__jki_lib_state_machine.vi"("State(s) in (\"\")"=w253) -> ("States Out"=w252:string)  [unwired: 14 in]
          }
          frame "Data: Clear Graphs" {
            w255 = cluster{"X":dbl, "Y":dbl}[] [] ("Graphs Data.SMU Data")
            n106 = Bundle By Name(cluster=w257, "Graphs Data.SMU Data"=w255, "Graphs Data.LIA Data"=w255, "Graphs Data.SMU Buffer"=w255, "Graphs Data.LIA Buffer"=w255) -> (w256:T14)
            n107 = call <vilib>:"Add State(s) to Queue__jki_lib_state_machine.vi"("State(s) in Front (\"\")"="Data: Initialize Grid" ("State(s) in Front (\"\")"), "State(s) in (\"\")"=w259) -> ("States Out"=w260:string)  [unwired: 13 in]
          }
          frame "Data: Clear Grid" {
            w268 = 0.0  # Initial Value
            n108 = Unbundle By Name(w266) -> ("X Count"=w262:i32, "Y Count"=w267:i32)
            n109 = Initialize Array(w268, w267, w262) -> (w264:dbl[][])
            n110 = Bundle By Name(cluster=w266, "Grid Data.SMU Image.Raw"=w264, "Grid Data.SMU Image.Normalized"=w264, "Grid Data.LIA Image.Raw"=w264, "Grid Data.LIA Image.Normalized"=w264, "Grid Data.Filled Row"=0) -> (w265:T14)
            n111 = call <vilib>:"Add State(s) to Queue__jki_lib_state_machine.vi"("State(s) in (\"\")"=w272) -> ("States Out"=w271:string)  [unwired: 14 in]
          }
          frame "---------- UI ----------" {
            # "Do not put any code in this frame.\n(It is a separator no-op. You can make a copy of this frame to create a new UI frame)"
            n112 = call <vilib>:"Add State(s) to Queue__jki_lib_state_machine.vi"("State(s) in (\"\")"=w277) -> ("States Out"=w276:string)  [unwired: 14 in]
          }
          frame "UI: Initialize" {
            w283 = T18 1 items=["Grayscale (U8)", "Grayscale (I16)", "Grayscale (SGL)", "Complex (CSG)", "RGB (U32)", "HSL (U32)", "RGB (U64)"] ("Image Type")
            w285 = T18 1 items=["Grayscale (U8)", "Grayscale (I16)", "Grayscale (SGL)", "Complex (CSG)", "RGB (U32)", "HSL (U32)", "RGB (U64)"] ("Image Type")
            w289 = T3."Disabled and Grayed Out" ("Disabled")
            # "Initialize the User Interface, here.\n(this is called automatically, by the Macro: Init)"
            n113 = property on="Start Button" class="Bool"("DisabledEnum"=w289) -> ()  [unwired: 2 in, 2 out]
            n114 = property on="Pause Button" class="Bool"("DisabledEnum"=w289) -> ()  [unwired: 2 in, 2 out]
            n115 = property on="Stop Button" class="Bool"("DisabledEnum"=w289) -> ()  [unwired: 2 in, 2 out]
            n116 = invoke on="Initialized" class="Bool (strict)" method="Reinit To Default"() -> ()  [unwired: 3 in, 3 out]
            n117 = call "IMAQ Create"("Image Name"="SMU I16 Image", "Image Type"=w285, "error in (no error)"=w280) -> ("New Image"=w282:T1, "error out"=w279:errorcluster)  [unwired: 2 in]
            n118 = call "IMAQ Create"("Image Name"="LIA I16 Image", "Image Type"=w283, "error in (no error)"=w279) -> ("New Image"=w281:T1, "error out"=w278:errorcluster)  [unwired: 2 in]
            n119 = Bundle By Name(cluster=w288, "SMU Image"=w282, "LIA Image"=w281) -> (w287:T14)
            n120 = call <vilib>:"Add State(s) to Queue__jki_lib_state_machine.vi"("State(s) in (\"\")"=w292) -> ("States Out"=w291:string)  [unwired: 14 in]
          }
          frame "UI: Cursor Set" {
            # "Argument"
            # "Initialize the User Interface, here.\n(this is called automatically, by the Macro: Init)"
            n121 = disable-structure shown="Default" {
              disable-tunnel: w295 -> [w300 w303]
              disable-tunnel: [w300 w302] -> w294
              disable-tunnel: w293 -> [_ w301]
              frame condition #0 {
              }
              frame condition #1 (active) {
                n122 = case shown="\"Idle\", Default" w301 {
                  tunnel: w303 -> [w305 w307]
                  tunnel: [w304 w306] -> w302
                  frame "Idle", Default {
                    n123 = call <vilib>:"Unset Busy.vi"("error in (no error)"=w305) -> ("error out"=w304:errorcluster)  [unwired: 10 in]
                  }
                  frame "Busy" {
                    n124 = call <vilib>:"Set Busy.vi"("error in (no error)"=w307) -> ("error out"=w306:errorcluster)  [unwired: 9 in, 1 out]
                  }
                }
              }
            }
            n125 = call <vilib>:"Add State(s) to Queue__jki_lib_state_machine.vi"("State(s) in (\"\")"=w299) -> ("States Out"=w298:string)  [unwired: 14 in]
          }
          frame "UI: Front Panel State" {
            # "Argument"
            # "Set Front Panel Open or Closed\n(Usage: \"UI: Front Panel State >> Open|Close\")"
            n126 = Unbundle By Name(w311) -> ("Core.Current VI Reference"=w310:refnum<vi>)
            n127 = disable-structure shown="Default" {
              disable-tunnel: w313 -> [w319 w342]
              disable-tunnel: [w318 w342] -> w312
              disable-tunnel: w310 -> [w317 _]
              disable-tunnel: w309 -> [w316 _]
              frame condition #0 (active) {
                n128 = case shown="\"Close\"" w316 {
                  tunnel: w319 -> [w323 w336]
                  tunnel: [w325 w337] -> w318
                  tunnel: w317 -> [w324 w334]
                  frame "Open", Default {
                    n129 = property class="VI"(reference=w324, error in=w323) -> (reference out=w321:refnum<vi>, error out=w322:errorcluster, "FP.State"=w320:T5)
                    n130 = case shown="\"Closed\"" w320 {
                      tunnel: [w328 w331] -> w325
                      tunnel: w322 -> [w327 w331]
                      tunnel: w321 -> [w326 _]
                      frame "Closed" {
                        n131 = invoke class="VI" method="FP.Open"(reference=w326, error in=w327, "Activate"=TRUE, "State"=T5."Standard") -> (error out=w328:errorcluster)  [unwired: 1 in, 4 out]
                      }
                      frame Default {
                      }
                    }
                  }
                  frame "Close" {
                    n132 = property class="VI"(reference=w334, error in=w336) -> (reference out=w333:refnum<vi>, error out=w335:errorcluster, "FP.State"=w332:T5)
                    n133 = case shown="Default" w332 {
                      tunnel: [w338 w341] -> w337
                      tunnel: w335 -> [w338 w340]
                      tunnel: w333 -> [_ w339]
                      frame "Invalid", "Closed" {
                      }
                      frame Default {
                        n134 = invoke class="VI" method="FP.Close"(reference=w339, error in=w340) -> (error out=w341:errorcluster)  [unwired: 1 in, 2 out]
                      }
                    }
                  }
                }
              }
              frame condition #1 {
              }
            }
            n135 = call <vilib>:"Add State(s) to Queue__jki_lib_state_machine.vi"("State(s) in (\"\")"=w315) -> ("States Out"=w314:string)  [unwired: 14 in]
          }
          frame "UI: Update Graphs" {
            n136 = Unbundle By Name(w345) -> ("Graphs Data.SMU Data"=→"SMU":cluster{"X":dbl, "Y":dbl}[], "Graphs Data.LIA Data"=→"LIA":cluster{"X":dbl, "Y":dbl}[])
            n137 = call <vilib>:"Add State(s) to Queue__jki_lib_state_machine.vi"("State(s) in (\"\")"=w349) -> ("States Out"=w348:string)  [unwired: 14 in]
          }
          frame "UI: Update Images" {
            n138 = Unbundle By Name(w352) -> ("SMU Image"=→"SMU":T1, "LIA Image"=→"LIA":T1)
            n139 = call <vilib>:"Add State(s) to Queue__jki_lib_state_machine.vi"("State(s) in (\"\")"=w356) -> ("States Out"=w355:string)  [unwired: 14 in]
          }
          frame "---------- Macro ----------" {
            # "Do not put any code in this frame.\n(It is a separator no-op. You can make a copy of this frame to create a new Macro frame)"
            n140 = call <vilib>:"Add State(s) to Queue__jki_lib_state_machine.vi"("State(s) in (\"\")"=w361) -> ("States Out"=w360:string)  [unwired: 14 in]
          }
          frame "Macro: Initialize" {
            w364 = "UI: Initialize\n//UI: Front Panel State >> Open"  # UI: Initialize //UI: Front Panel State >> Open
            # "Initialization Macro\n(This is called once, when the VI starts)"
            n141 = call <vilib>:"Add State(s) to Queue__jki_lib_state_machine.vi"("State(s) in Front (\"\")"="Data: Initialize\nInitialize Core Data\nEvents: Register", "State(s) in (\"\")"="Process: Sync", "State(s) at Back (\"\")"=w364) -> ("States Out"=w363:string)  [unwired: 12 in]
            n142 = call <vilib>:"Add State(s) to Queue__jki_lib_state_machine.vi"("State(s) in Front (\"\")"=w363, "State(s) in (\"\")"=w370) -> ("States Out"=w369:string)  [unwired: 13 in]
          }
          frame "Macro: Exit" {
            # "Exit Macro\n(This is called once, when the VI exits)"
            n143 = Unbundle By Name(w375) -> ("Core.Close Panel on Exit?"=w381:bool)
            n144 = Select(t="//UI: Front Panel State >> Close", s=w381, f="") -> (s? t:f=w378:string)
            n145 = call <vilib>:"Add State(s) to Queue__jki_lib_state_machine.vi"("State(s) in Front (\"\")"="Data: Cleanup\nEvents: Unregister", "State(s) in (\"\")"="Process: Sync", "State(s) at Back (\"\")"="Exit") -> ("States Out"=w372:string)  [unwired: 12 in]
            n146 = call <vilib>:"Add State(s) to Queue__jki_lib_state_machine.vi"("State(s) in (\"\")"=w378, "State(s) at Back (\"\")"=w372) -> ("States Out"=w377:string)  [unwired: 13 in]
            n147 = call <vilib>:"Add State(s) to Queue__jki_lib_state_machine.vi"("State(s) in Front (\"\")"=w377, "State(s) in (\"\")"=w384) -> ("States Out"=w383:string)  [unwired: 13 in]
          }
          frame "Macro: Update Grid" {
            n148 = call <vilib>:"Add State(s) to Queue__jki_lib_state_machine.vi"("State(s) in Front (\"\")"="Action: Grid Data Calculate Min/Max\nAction: Grid Data Normalize\nAction: Grid Data Create Images\nUI: Update Images" ("t"), "State(s) in (\"\")"=w390) -> ("States Out"=w389:string)  [unwired: 13 in]
          }
          frame "Macro: Data Clear" {
            n149 = call <vilib>:"Add State(s) to Queue__jki_lib_state_machine.vi"("State(s) in Front (\"\")"="Data: Clear Graphs\nData: Clear Grid" ("t"), "State(s) in (\"\")"=w396) -> ("States Out"=w395:string)  [unwired: 13 in]
          }
          frame "Macro: Update UI" {
            n150 = call <vilib>:"Add State(s) to Queue__jki_lib_state_machine.vi"("State(s) in Front (\"\")"="UI: Update Graphs\nMacro: Update Grid" ("t"), "State(s) in (\"\")"=w402) -> ("States Out"=w401:string)  [unwired: 13 in]
          }
          frame "---------- Process ----------" {
            # "Template Separator\n(You can make a copy of, or modify, this frame)"
            n151 = call <vilib>:"Add State(s) to Queue__jki_lib_state_machine.vi"("State(s) in (\"\")"=w407) -> ("States Out"=w406:string)  [unwired: 14 in]
          }
          frame "Process: Sync" {
            n152 = Unbundle By Name(w415) -> ("Self Reference"=w411:refnum<class "Measurement.PhotocurrentMapping.UI.lvclass">)
            n153 = call <vilib>:"WaitOnProcessSync.vi"("error in (no error)"=w410, "SMO"=w411) -> ("error out"=w409:errorcluster, "Don't run?"=w414:bool)  [unwired: 7 in, 1 out]
            n154 = Select(t="Data: Cleanup\nEvents: Unregister\nExit", s=w414, f="") -> (s? t:f=w408:string)
            n155 = call <vilib>:"Add State(s) to Queue__jki_lib_state_machine.vi"("State(s) in Front (\"\")"=w408, "State(s) in (\"\")"=w418) -> ("States Out"=w417:string)  [unwired: 13 in]
          }
          frame "---------- Events ----------" {
            # "Template Separator\n(You can make a copy of, or modify, this frame)"
            n156 = call <vilib>:"Add State(s) to Queue__jki_lib_state_machine.vi"("State(s) in (\"\")"=w423) -> ("States Out"=w422:string)  [unwired: 14 in]
          }
          frame "Events: Register" {
            # "Measurement base class Public Events"
            # "Base Class Protected Events"
            n157 = Unbundle By Name(w429) -> ("Dependencies.Measurement.PhotocurrentMapping"=w428:refnum<class "Measurement.PhotocurrentMapping.lvclass">)
            n158 = Unbundle By Name(w429) -> ("Self Reference"=w434:refnum<class "Measurement.PhotocurrentMapping.UI.lvclass">)
            n159 = call <vilib>:"GetProtectedEvents.vi"("SMO"=w434) -> ("error out"=w430:errorcluster, "SMO Protected Events"=w435:T19)  [unwired: 8 in, 1 out]
            n160 = call "Measurement.GetPublicEventsRegistration.vi"("Measurement in"=w428) -> ("error out"=w424:errorcluster, "Measurement Public Events"=w425:refnum<event-registration>)  [unwired: 8 in, 1 out]
            n161 = register-events(w435) -> (reference out=w427:refnum<event-registration>, error out=w432:errorcluster)  [unwired: 2 in]
            n162 = Bundle("Event Registration Refnum"=w427, "Measurement Public Events"=w425) -> (w426:T20)  [unwired: 1 in]
            n163 = Merge Errors(w433, w432, w430, w424) -> (w431:errorcluster)
            n164 = call <vilib>:"Add State(s) to Queue__jki_lib_state_machine.vi"("State(s) in (\"\")"=w437) -> ("States Out"=w436:string)  [unwired: 14 in]
          }
          frame "Events: Unregister" {
            n165 = Unregister For Events(event registration refnum=w440, error in=w439) -> (error out=w438:errorcluster)
            n166 = call <vilib>:"Add State(s) to Queue__jki_lib_state_machine.vi"("State(s) in (\"\")"=w443) -> ("States Out"=w442:string)  [unwired: 14 in]
          }
          frame "---------- Action ----------" {
            n167 = Unbundle By Name(w446) -> ("Self Reference"=w444:refnum<class "Measurement.PhotocurrentMapping.UI.lvclass">)
            n168 = Bundle By Name(cluster=w446, "Self Reference"=w444) -> (w445:T14)
            n169 = call <vilib>:"Add State(s) to Queue__jki_lib_state_machine.vi"("State(s) in (\"\")"=w450) -> ("States Out"=w449:string)  [unwired: 14 in]
          }
          frame "Action: Notify UI Closed" {
            # "Notify that the UI has been closed"
            n170 = Unbundle By Name(w453) -> ("Self Reference"=w454:refnum<class "Measurement.PhotocurrentMapping.UI.lvclass">)
            n171 = call <vilib>:"Hide.vi"("error in (no error)"=w452, "SMO.UI"=w454) -> ("error out"=w451:errorcluster)  [unwired: 8 in, 1 out]
            n172 = call <vilib>:"Add State(s) to Queue__jki_lib_state_machine.vi"("State(s) in (\"\")"=w457) -> ("States Out"=w456:string)  [unwired: 14 in]
          }
          frame "Action: Measured Processing" {
            n173 = call <vilib>:"Add State(s) to Queue__jki_lib_state_machine.vi"("State(s) in Front (\"\")"="Action: Graphs Data Add New\nAction: Grid Data Add New", "State(s) in (\"\")"=w463) -> ("States Out"=w462:string)  [unwired: 13 in]
          }
          frame "Action: Graphs Data Add New" {
            n174 = Unbundle By Name(w476) -> ("Graphs Data.SMU Buffer"=w473:cluster{"X":dbl, "Y":dbl}[], "Graphs Data.LIA Buffer"=w472:cluster{"X":dbl, "Y":dbl}[], "Measured"=w477:T10)
            n175 = Unbundle By Name(w477) -> ("X Value, units"=w470:dbl, "Current, A"=w471:dbl, "Magnitude"=w469:dbl, "Last Row Element?"=w466:bool)
            n176 = Bundle("X Value, units"=w470, "Current, A"=w471) -> (w468:cluster{"X Value, units":dbl, "Current, A":dbl})  [unwired: 1 in]
            n177 = Bundle("X Value, units"=w470, "Magnitude"=w469) -> (w467:cluster{"X Value, units":dbl, "Magnitude":dbl})  [unwired: 1 in]
            n178 = Build Array (concatenate)(w473, w468) -> (w464:T21)
            n179 = Build Array (concatenate)(w472, w467) -> (w465:cluster{"X Value, units":dbl, "Magnitude":dbl}[])
            n180 = case shown="True" w466 {
              tunnel: w476 -> [w485 w491]
              tunnel: [w484 w490] -> w475
              tunnel: [_ "UI: Update Graphs"] -> w474
              tunnel: w465 -> [w482 w487]
              tunnel: w464 -> [w483 w488]
              frame False {
                n181 = Bundle By Name(cluster=w485, "Graphs Data.SMU Buffer"=w483, "Graphs Data.LIA Buffer"=w482) -> (w484:T14)
              }
              frame True {
                w486 = cluster{"X":dbl, "Y":dbl}[] [] ("Graphs Data.SMU Buffer")
                # "Clear buffer arrays"
                # "Copy collected data to arrays for display on graphs"
                n182 = Bundle By Name(cluster=w491, "Graphs Data.SMU Data"=w488, "Graphs Data.LIA Data"=w487, "Graphs Data.SMU Buffer"=w486, "Graphs Data.LIA Buffer"=w486) -> (w490:T14)
              }
            }
            n183 = call <vilib>:"Add State(s) to Queue__jki_lib_state_machine.vi"("State(s) in Front (\"\")"=w474, "State(s) in (\"\")"=w481) -> ("States Out"=w480:string)  [unwired: 13 in]
          }
          frame "Action: Grid Data Add New" {
            n184 = Unbundle By Name(w507) -> ("Grid Data.SMU Image.Raw"=w508:dbl[][], "Grid Data.LIA Image.Raw"=w502:dbl[][], "Measured"=w505:T10, "Grid Data.Filled Row"=w493:i32)
            n185 = Unbundle By Name(w505) -> ("X Index"=w504:i32, "Y Index"=w503:i32, "Current, A"=w501:dbl, "Magnitude"=w500:dbl, "Last Row Element?"=w494:bool)
            n186 = case shown="True" w494 {
              tunnel: w493 -> [w513 w515]
              tunnel: [w513 w514] -> w492
              frame False {
              }
              frame True {
                n187 = Increment(x=w515) -> (x+1=w514:i32)
              }
            }
            n188 = Replace Array Subset(array=w508, new element=w501, index (row)=w503, index (col)=w504) -> (w499:dbl[][])
            n189 = Replace Array Subset(array=w502, new element=w500, index (row)=w503, index (col)=w504) -> (w498:dbl[][])
            n190 = Bundle By Name(cluster=w507, "Grid Data.SMU Image.Raw"=w499, "Grid Data.LIA Image.Raw"=w498, "Grid Data.Filled Row"=w492) -> (w506:T14)
            n191 = Select(t="Macro: Update Grid", s=w494, f="") -> (s? t:f=w495:string)
            n192 = call <vilib>:"Add State(s) to Queue__jki_lib_state_machine.vi"("State(s) in Front (\"\")"=w495, "State(s) in (\"\")"=w512) -> ("States Out"=w511:string)  [unwired: 13 in]
          }
          frame "Action: Grid Data Calculate Min/Max" {
            n193 = property on="SMU Auto Scale" class="Bool (strict)"() -> ("Value"=w522:bool)  [unwired: 2 in, 2 out]
            n194 = property on="LIA Auto Scale" class="Bool (strict)"() -> ("Value"=w519:bool)  [unwired: 2 in, 2 out]
            n195 = case shown="True" w522 {
              tunnel: [w536 w538] -> w521
              tunnel: [w535 w537] -> w520
              tunnel: w518 -> [_ w541]
              frame False {
                n196 = property on="SMU minimum, A" class="DigNum (strict)"() -> ("Value"=w536:dbl)  [unwired: 2 in, 2 out]
                n197 = property on="SMU maximum, A" class="DigNum (strict)"() -> ("Value"=w535:dbl)  [unwired: 2 in, 2 out]
              }
              frame True {
                n198 = Unbundle By Name(w541) -> ("Grid Data.SMU Image.Raw"=w540:dbl[][], "Grid Data.Filled Row"=w539:i32)
                n199 = call "2D Array Min Max.vi"("Rows Include"=w539, "Array"=w540) -> ("min value"=w538:dbl, "max value"=w537:dbl)
                n200 = property on="SMU minimum, A" class="DigNum (strict)"("Value"=w538) -> ()  [unwired: 2 in, 2 out]
                n201 = property on="SMU maximum, A" class="DigNum (strict)"("Value"=w537) -> ()  [unwired: 2 in, 2 out]
              }
            }
            n202 = case shown="True" w519 {
              tunnel: [w529 w531] -> w517
              tunnel: [w528 w530] -> w516
              tunnel: w518 -> [_ w534]
              frame False {
                n203 = property on="LIA minimum" class="DigNum (strict)"() -> ("Value"=w529:dbl)  [unwired: 2 in, 2 out]
                n204 = property on="LIA maximum" class="DigNum (strict)"() -> ("Value"=w528:dbl)  [unwired: 2 in, 2 out]
              }
              frame True {
                n205 = Unbundle By Name(w534) -> ("Grid Data.LIA Image.Raw"=w533:dbl[][], "Grid Data.Filled Row"=w532:i32)
                n206 = call "2D Array Min Max.vi"("Rows Include"=w532, "Array"=w533) -> ("min value"=w531:dbl, "max value"=w530:dbl)
                n207 = property on="LIA minimum" class="DigNum (strict)"("Value"=w531) -> ()  [unwired: 2 in, 2 out]
                n208 = property on="LIA maximum" class="DigNum (strict)"("Value"=w530) -> ()  [unwired: 2 in, 2 out]
              }
            }
            n209 = Bundle By Name(cluster=w518, "Grid Data.SMU Image.Minimum"=w521, "Grid Data.SMU Image.Maximum"=w520, "Grid Data.LIA Image.Minimum"=w517, "Grid Data.LIA Image.Maximum"=w516) -> (w523:T14)
            n210 = call <vilib>:"Add State(s) to Queue__jki_lib_state_machine.vi"("State(s) in (\"\")"=w527) -> ("States Out"=w526:string)  [unwired: 14 in]
          }
          frame "Action: Grid Data Normalize" {
            n211 = Unbundle By Name(w542) -> ("Grid Data.SMU Image.Raw"=w552:dbl[][], "Grid Data.SMU Image.Minimum"=w550:dbl, "Grid Data.SMU Image.Maximum"=w549:dbl)
            n212 = Unbundle By Name(w542) -> ("Grid Data.LIA Image.Raw"=w544:dbl[][], "Grid Data.LIA Image.Minimum"=w545:dbl, "Grid Data.LIA Image.Maximum"=w546:dbl)
            n213 = call "2D Array Normalize.vi"("Factor"=1024, "Maximum"=w549, "Minimum"=w550, "Array in"=w552) -> ("Array out"=w551:dbl[][])  [unwired: 7 in]
            n214 = call "2D Array Normalize.vi"("Factor"=1024, "Maximum"=w546, "Minimum"=w545, "Array in"=w544) -> ("Array out"=w543:dbl[][])  [unwired: 7 in]
            n215 = Bundle By Name(cluster=w542, "Grid Data.SMU Image.Normalized"=w551, "Grid Data.LIA Image.Normalized"=w543) -> (w553:T14)
            n216 = call <vilib>:"Add State(s) to Queue__jki_lib_state_machine.vi"("State(s) in (\"\")"=w557) -> ("States Out"=w556:string)  [unwired: 14 in]
          }
          frame "Action: Grid Data Create Images" {
            n217 = Unbundle By Name(w563) -> ("SMU Image"=w569:T1, "Grid Data.SMU Image.Normalized"=w568:dbl[][])
            n218 = Unbundle By Name(w563) -> ("LIA Image"=w565:T1, "Grid Data.LIA Image.Normalized"=w564:dbl[][])
            n219 = call "IMAQ ArrayToImage"("error in (no error)"=w561, "Image Pixels (I16)"=w568, "Image"=w569) -> ("error out"=w559:errorcluster, "Image Out"=w567:T1)  [unwired: 7 in]
            n220 = call "IMAQ ArrayToImage"("error in (no error)"=w561, "Image Pixels (I16)"=w564, "Image"=w565) -> ("error out"=w558:errorcluster, "Image Out"=w562:T1)  [unwired: 7 in]
            n221 = Bundle By Name(cluster=w563, "SMU Image"=w567, "LIA Image"=w562) -> (w566:T14)
            n222 = Merge Errors(w559, w558) -> (w560:errorcluster)
            n223 = call <vilib>:"Add State(s) to Queue__jki_lib_state_machine.vi"("State(s) in (\"\")"=w572) -> ("States Out"=w571:string)  [unwired: 14 in]
          }
        }
      }
    }
    frame Error {
    }
  }
  n224 = call-parent "Process.vi"("error in (no error)"=w8, "SMO.UI"=w7) -> ("error out"=w5:errorcluster, "SMO.UI out"=→"Measurement.WavelengthSweeping.UI out":refnum<class "Measurement.PhotocurrentMapping.UI.lvclass">)  [unwired: 8 in]
  n225 = Merge Errors(w5, w4) -> (→"error out":errorcluster)
